vi "Thermometer.vi"(1 "Temp Scale":bool) -> (0 "Temperature":dbl(slide) scale=0.0..100.0)   [LabVIEW 2018]
panel:
  # "Deg C"
  # "Deg F"
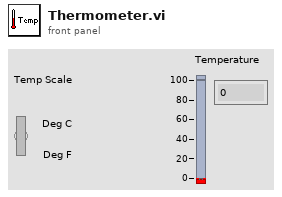
[diagram p1: front panel]
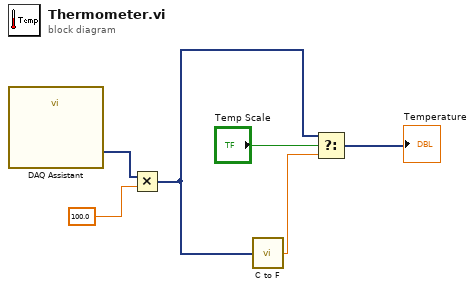
[diagram p0: block diagram]
diagram:
  n1 = call "DAQ Assistant"() -> ("data"=w6:dynamicdata)  [unwired: 17 in, 2 out]
  n2 = Multiply(x=w6, y=100.0) -> (x*y=w4:dynamicdata)
  n3 = call "C to F.vi"("deg C"=w4) -> ("deg F"=w3:dbl)
  n4 = Select(t=w4, s="Temp Scale", f=w3) -> (s? t:f=→"Temperature":dynamicdata)
